vi "velocity-number-in-counts-per-sec.vi"(9 "Axis Select":u8(slide)=1 min=1 max=4 step=1 scale=1.0..4.0, 10 "unit":T1(ring), 11 "velocity":dbl) -> (1 "unit":string, 3 "counts":dbl format="%#_18f")   [LabVIEW 2009]
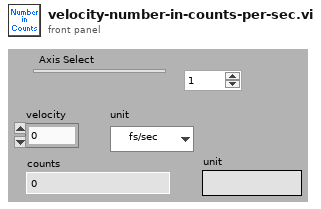
[diagram p1: front panel]
types:
  T1 = enum16{"fs/sec", "ps/sec", "um/sec", "mm/sec", "counts/sec"}
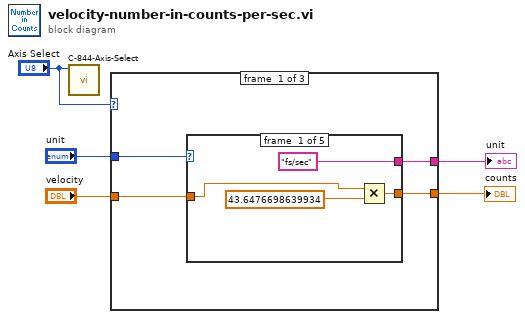
[diagram p0: block diagram]
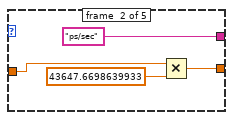
[diagram p2: hidden frame]
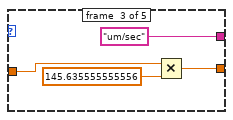
[diagram p3: hidden frame]
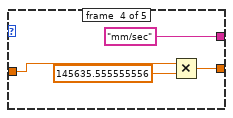
[diagram p4: hidden frame]
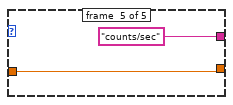
[diagram p5: hidden frame]
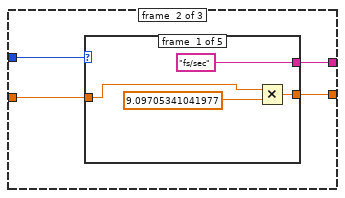
[diagram p6: hidden frame]
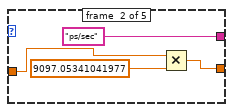
[diagram p7: hidden frame]
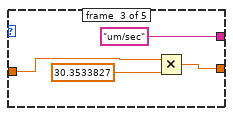
[diagram p8: hidden frame]
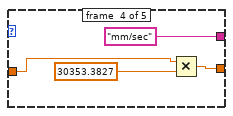
[diagram p9: hidden frame]
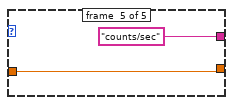
[diagram p10: hidden frame]
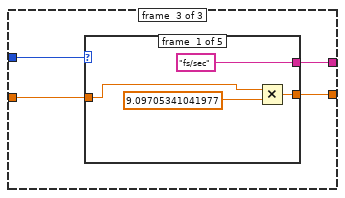
[diagram p11: hidden frame]
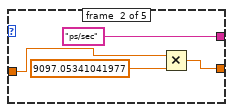
[diagram p12: hidden frame]
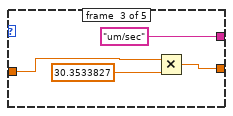
[diagram p13: hidden frame]
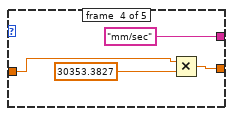
[diagram p14: hidden frame]
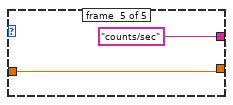
[diagram p15: hidden frame]
diagram:
  n1 = call "C-844-Axis-Select.vi"("Axis Select"="Axis Select") -> ()  [unwired: 9 in, 2 out]
  n2 = case shown="1, Default" "Axis Select" {
    tunnel: "velocity" -> [w7 w31 w53]
    tunnel: "unit" -> [w6 w30 w52]
    tunnel: [w8 w29 w50] -> w3
    tunnel: [w9 w28 w51] -> w2
    frame #0 {
      n3 = case shown="\"fs/sec\"" w6 {
        tunnel: w7 -> [w11 w15 w19 w23 w27]
        tunnel: [w13 w17 w21 w25 w27] -> w8
        tunnel: ["fs/sec" "ps/sec" "um/sec" "mm/sec" "counts/sec"] -> w9
        frame #0 {
          n4 = Multiply(x=w11, y=43.6476698639934) -> (x*y=w13:dbl)
        }
        frame #1 {
          n5 = Multiply(x=w15, y=43647.6698639933) -> (x*y=w17:dbl)
        }
        frame #2 {
          n6 = Multiply(x=w19, y=145.635555555556) -> (x*y=w21:dbl)
        }
        frame #3 {
          n7 = Multiply(x=w23, y=145635.555555556) -> (x*y=w25:dbl)
        }
        frame #4 {
        }
      }
    }
    frame #1 {
      n8 = case shown="\"fs/sec\"" w30 {
        tunnel: w31 -> [w33 w37 w41 w45 w49]
        tunnel: [w35 w39 w43 w47 w49] -> w29
        tunnel: ["fs/sec" "ps/sec" "um/sec" "mm/sec" "counts/sec"] -> w28
        frame #0 {
          n9 = Multiply(x=w33, y=9.09705341041977) -> (x*y=w35:dbl)
        }
        frame #1 {
          n10 = Multiply(x=w37, y=9097.05341041977) -> (x*y=w39:dbl)
        }
        frame #2 {
          n11 = Multiply(x=w41, y=30.3533827) -> (x*y=w43:dbl)
        }
        frame #3 {
          n12 = Multiply(x=w45, y=30353.3827) -> (x*y=w47:dbl)
        }
        frame #4 {
        }
      }
    }
    frame #2 {
      n13 = case shown="\"fs/sec\"" w52 {
        tunnel: w53 -> [w55 w59 w63 w67 w71]
        tunnel: [w57 w61 w65 w69 w71] -> w50
        tunnel: ["fs/sec" "ps/sec" "um/sec" "mm/sec" "counts/sec"] -> w51
        frame #0 {
          n14 = Multiply(x=w55, y=9.09705341041977) -> (x*y=w57:dbl)
        }
        frame #1 {
          n15 = Multiply(x=w59, y=9097.05341041977) -> (x*y=w61:dbl)
        }
        frame #2 {
          n16 = Multiply(x=w63, y=30.3533827) -> (x*y=w65:dbl)
        }
        frame #3 {
          n17 = Multiply(x=w67, y=30353.3827) -> (x*y=w69:dbl)
        }
        frame #4 {
        }
      }
    }
  }
  "counts" <- w3
  "unit" <- w2
